vi "Remove Duplicates from 1D Array (String)__ogtk.vi"(0 "Input Array":string[](array[string])) -> (1 "Output Array":string[](array[string]), 2 "indices of removed elements":i32[](array[numeric]))   [LabVIEW 2014, in "ZLIB.lvlib"]
doc: "This polymorphic VI removes all duplicate elements in <B>Input Array</B> and outputs the result as <B>Output Array</B>. It also outputs the <B>indices of removed elements<B>."
uses:
  ZLIB.lvlib
panel:
  # "Remove Duplicates from 1D Array.vi\n\nRemoves duplicate array elements and returns the indices of the removed elements\n\nPlease visit http://www.OpenG.org to learn about the\nOpen Source LabVIEW software movement.\n\nNOTICE -- YOU MUST LEAVE THIS NOTICE IN PLACE.  PER THE TERMS OF THE LICENSE BELOW, YOU MAY SUBLICENSE THIS SOFTWARE \nIN ANY WAY THAT DOES NOT CONFLICT WITH THIS LICENSE.\n\n### BSD License (http://www.opensource.org/licenses/bsd-license.php) Begin ###\n \nCopyright (c) 2002, Jim Kring <jim@jimkring.com>\n\nAll rights reserved.\n\nRedistribution and use in source and binary forms, with or without modification, are permitted provided that the following conditions are met:\n\n    * Redistributions of source code must retain the above copyright notice, this list of conditions and the following disclaimer.\n    * Redistributions in binary form must reproduce the above copyright notice, this list of conditions and the following disclaimer in the \n       documentation and/or other materials provided with the distribution.\n    * Neither the name of SciWare, James Kring, Inc., nor the names of its contributors may be used to endorse or promote products derived \n       from this software without specific prior written permission.\n\nTHIS SOFTWARE IS PROVIDED BY THE COPYRIGHT HOLDERS AND CONTRIBUTORS \"AS IS\" AND ANY EXPRESS OR IMPLIED WARRANTIES, \nINCLUDING, BUT NOT LIMITED TO, THE IMPLIED WARRANTIES OF MERCHANTABILITY AND FITNESS FOR A PARTICULAR PURPOSE ARE \nDISCLAIMED. IN NO EVENT SHALL THE COPYRIGHT OWNER OR CONTRIBUTORS BE LIABLE FOR ANY DIRECT, INDIRECT, INCIDENTAL,\n SPECIAL, EXEMPLARY, OR CONSEQUENTIAL DAMAGES (INCLUDING, BUT NOT LIMITED TO, PROCUREMENT OF SUBSTITUTE GOODS OR \nSERVICES; LOSS OF USE, DATA, OR PROFITS; OR BUSINESS INTERRUPTION) HOWEVER CAUSED AND ON ANY THEORY OF LIABILITY, \nWHETHER IN CONTRACT, STRICT LIABILITY, OR TORT (INCLUDING NEGLIGENCE OR OTHERWISE) ARISING IN ANY WAY OUT OF THE USE \nOF THIS SOFTWARE, EVEN IF ADVISED OF THE POSSIBILITY OF SUCH DAMAGE.\n\n### BSD License End ###"
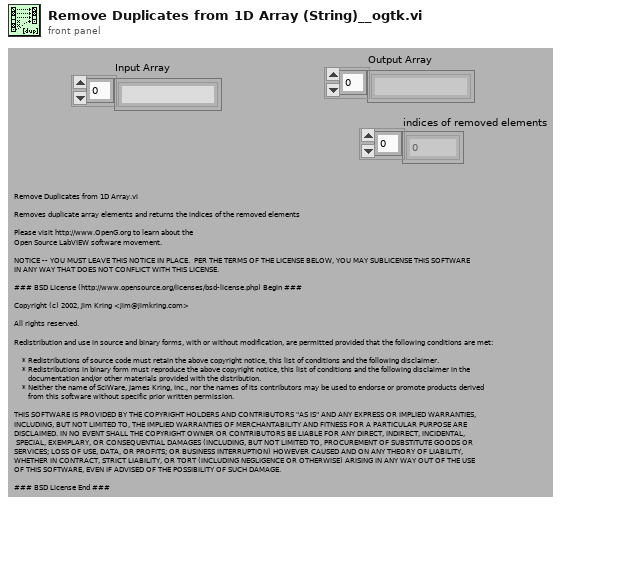
[diagram p1: front panel]
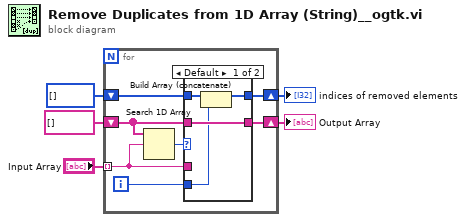
[diagram p0: block diagram]
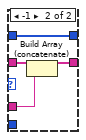
[diagram p2: hidden frame]
diagram:
  n1 = for {
    tunnel: "Input Array" -> [w11] mode=indexing
    shift-right: [w10] -> w3
    shift-left: string[] [] -> [w9]
    shift-right: [w7] -> w1
    shift-left: i32[] [] -> [w6]
    i -> [w8]
    n2 = Search 1D Array(1D array=w9, element=w11) -> (index of element=w12:i32)  [unwired: 1 in]
    n3 = case shown="Default" w12 {
      tunnel: w11 -> [_ w20]
      tunnel: [w16 w18] -> w10
      tunnel: w9 -> [w16 w19]
      tunnel: w8 -> [w13 _]
      tunnel: [w14 w17] -> w7
      tunnel: w6 -> [w15 w17]
      frame Default {
        n4 = Build Array (concatenate)(w15, w13) -> (w14:i32[])
      }
      frame -1 {
        n5 = Build Array (concatenate)(w19, w20) -> (w18:string[])
      }
    }
  }
  "Output Array" <- w3
  "indices of removed elements" <- w1
